vi "Close File.vi"(8 "error in (no error)":errorcluster, 11 "file_id":i32) -> (0 "error out":errorcluster)   [LabVIEW 2014, in "HDF5Tools.lvlib"]
uses:
  HDF5Tools.lvlib
  Release/HDF5Tools.dll
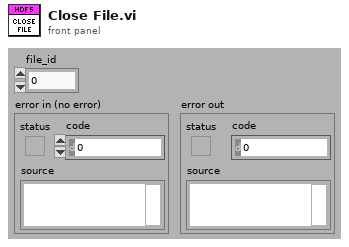
[diagram p1: front panel]
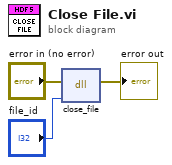
[diagram p0: block diagram]
diagram:
  n1 = dll-call lib="Z:/users/Manolis/Labview/Cajal/private/HDF5Tools32/Release/HDF5Tools.dll" fn="close_file"(error in="error in (no error)", "file_id"="file_id") -> (error out=→"error out":errorcluster)  [unwired: 4 in, 1 out]
